vi "Tmp_M submodule.vi"(9 "timeout ms":i32=1000) -> (0 "Error Out":errorcluster, 3 "Temperatures":T2[](array[typedef]) {"Time stamp" format="%<%H:%M:%S%2u\n%Y/%m/%d>T"})   [LabVIEW 2021, in "Temperature monitor.lvlib"]
doc: "Magnet module controls: power supply unit (PSU/SMS) and temperature monitor (TM/LSC218).\nPSU controls mainly: switch heater and ramping of current which runs throught coil.\nTM controls temperature of switch, coil and cryostat.\nMessage for magnet is a cluster that contains: {(enum) Command , (variant) Data}\nFor simplifieing of documentation, the Command is noted as a name of instruction, and Data is represented by a requered datatype (mostly cluster) name.\nCommands:\nInitialize(Magnet Config Constants) - Sugesstion: Load configuration constants from configuration file.\nSet field (Set field{B, R, cr}) - B-field[T], R-ramp[A/s], cr - custom ramp[bool].\nSwitch mode(mode) - to persistant, or to ramping.\nBlackout() - undone functionality of emergency deenergizing.\nUpdate() - Important! This triggers update of data from instruments. Shoud occure in regular intervals as priority message.\nResponses:\nMagnet initialized ();\nTM revision(temperature monitor revision);\nMagnet init error(error);\nSetting field(Set Field{B, R, cr});\nWarning(string);\nSwitching to(mode);\nUpdate error(error);\nTM update(TM sensors);\nPSU update(PSU data);\nMagnet status();"
uses:
  submodules/Temperature monitor/Temperature monitor.lvlib
  ctl/Cryostat temperature sensors.ctl
  Magnet module.lvlib
  Messenger service/Data types/Module name.ctl
  Messenger service/MessengerLib.lvlib
  ctl/TM states.ctl
  <userlib>/Queued messenger lib/Queued messenger.lvlib
  <userlib>/Queued messenger lib/TypeDefs/Mailbox ref.ctl
  submodules/Temperature monitor/Typedefs/TM_status.ctl
  <vilib>/WebDAVClient/NI_WebDAV.lvlib
panel:
  in  "Instr VISA ref":refnum<visa-resource-name>
  in  "This mailbox":T1
  in  "Supra mailbox":T1
  out "Connected":bool
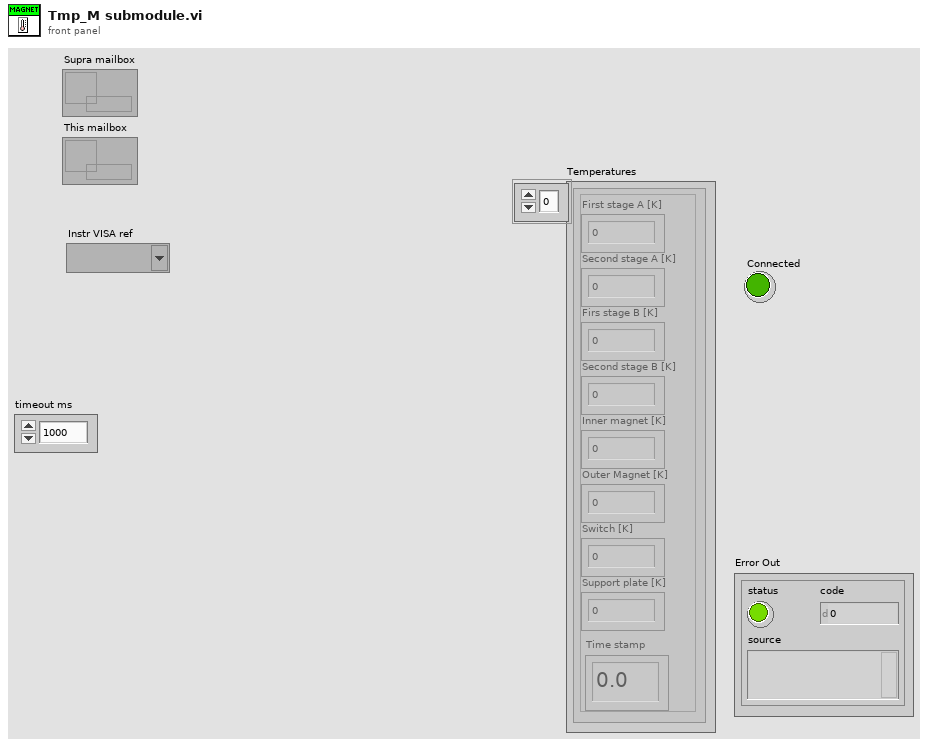
[diagram p1: front panel]
types:
  T1 = typedef "Queued messenger.lvlib/Mailbox ref.ctl" = refnum<queue>
  T2 = typedef "Magnet module.lvlib/Cryostat temperature sensors.ctl" = cluster{"First stage A [K]":dbl, "Second stage A [K]":dbl, "Firs stage B [K]":dbl, "Second stage B [K]":dbl, "Inner magnet [K]":dbl, "Outer Magnet [K]":dbl, "Switch [K]":dbl, "Support plate [K]":dbl, "Time stamp":dbl}
  T3 = typedef "TM_status.ctl" = cluster{"Supramodule":T1, "This module":T1, "Standalone?":bool, "Stopped?":bool, "Instr VISA ref":refnum<visa-resource-name>, "Connected?":bool}
  T4 = typedef "TM states.ctl" = enum16{"Initialize", "Wait for event", "Check message", "End"}
  T5 = typedef "MessengerLib.lvlib/Module name.ctl" = enum16{"Emty", "Magnet", "VTI", "Excitation", "Servo", "Acquisition", "Rotator", "Digitizer", "SMU2450", "Carousel", "Multimeter", "Tmp monitor", "Power monitor"}
  T6 = enum32{"Bad", "Idle", "Run top level", "Running"}
  T7 = typedef "Temperature monitor.lvlib/Tmp_M commands.ctl" = enum16{"Ignore", "Connect", "Set timeout", "Update", "Disconnect"}
  T8 = typedef "MessengerLib.lvlib/Mailbox address.ctl" = refnum<queue>
  T9 = typedef "Temperature monitor.lvlib/TM Revision.ctl" = cluster{"Instr Serial Number":string, "Instr Driver Revision":string, "Instr Firmware Revision":string, "Instr Model Number":string}
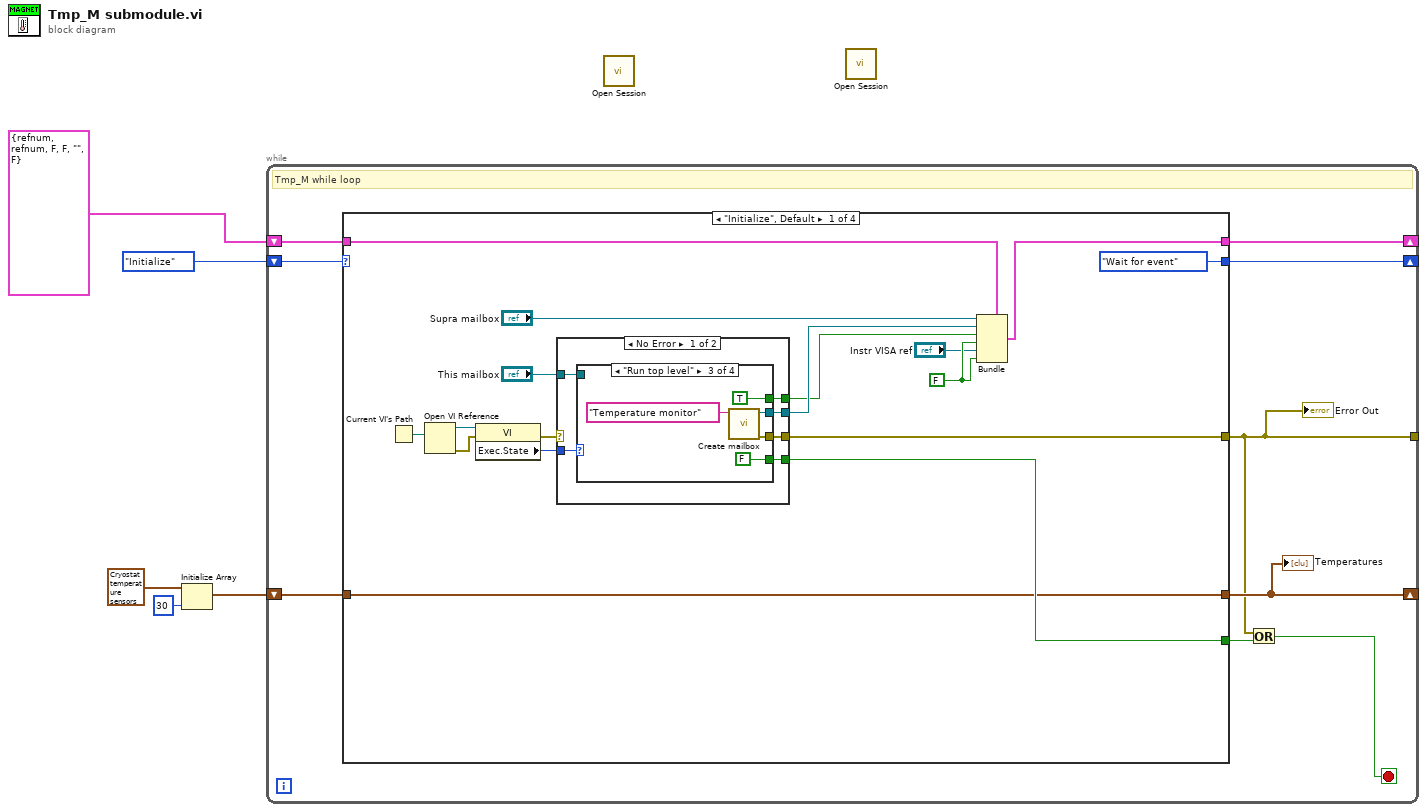
[diagram p0: block diagram]
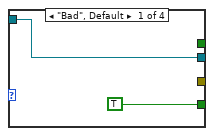
[diagram p2: hidden frame]
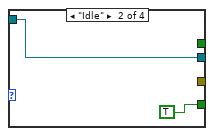
[diagram p3: hidden frame]
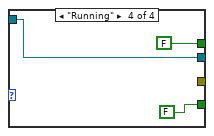
[diagram p4: hidden frame]
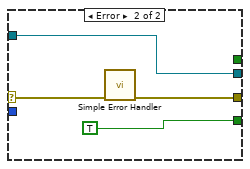
[diagram p5: hidden frame]
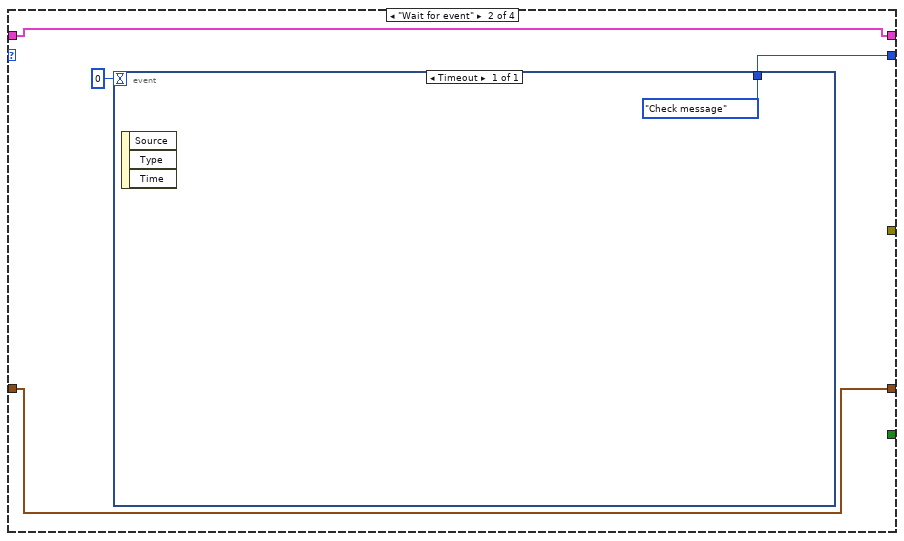
[diagram p6: hidden frame]
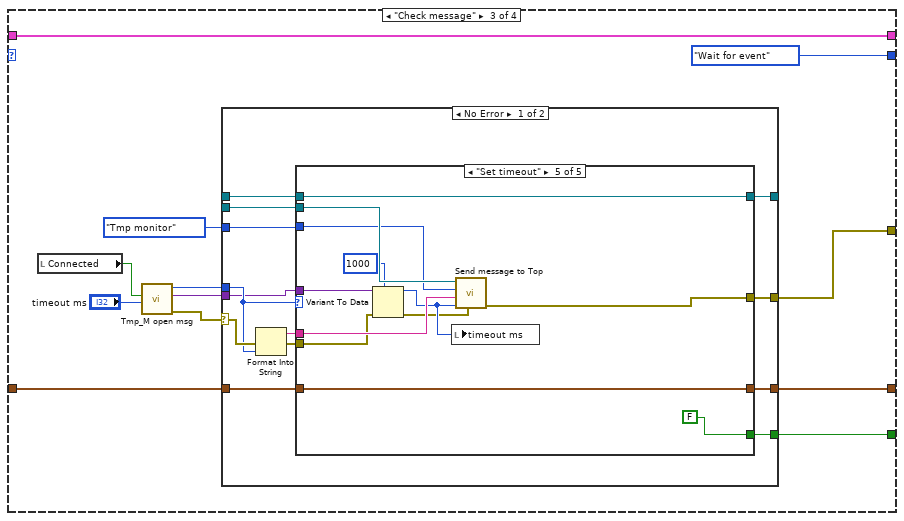
[diagram p7: hidden frame]
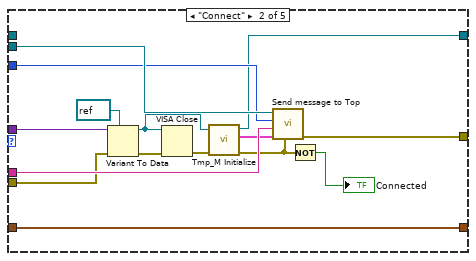
[diagram p9: hidden frame]
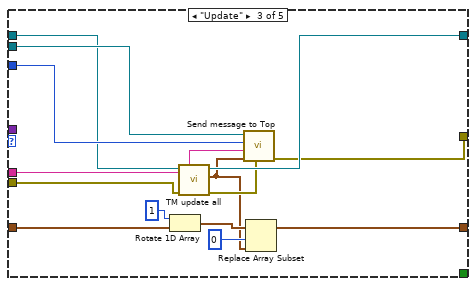
[diagram p10: hidden frame]
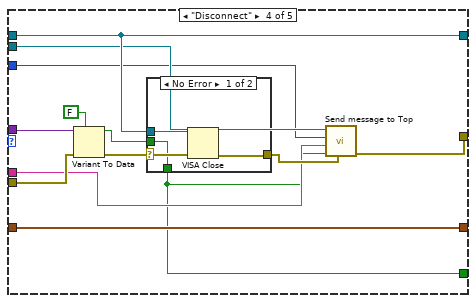
[diagram p11: hidden frame]
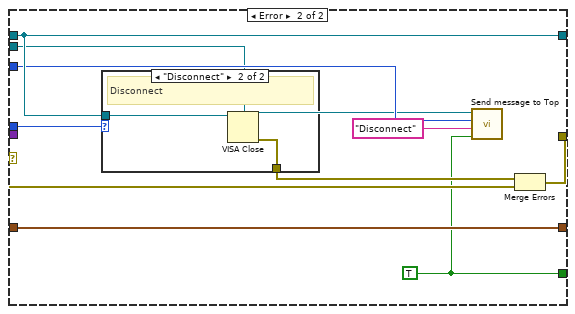
[diagram p13: hidden frame]
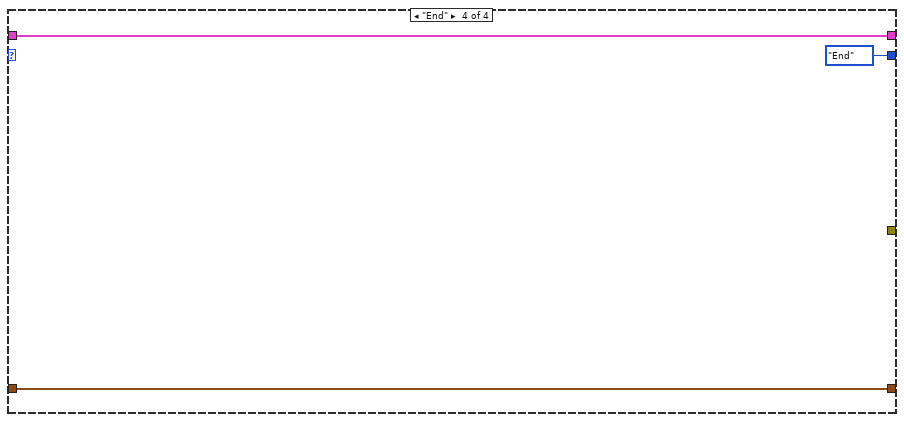
[diagram p15: hidden frame]
diagram:
  n1 = Initialize Array(T2 {"First stage A [K]"=0.0, "Second stage A [K]"=0.0, "Firs stage B [K]"=0.0, "Second stage B [K]"=0.0, "Inner magnet [K]"=0.0, "Outer Magnet [K]"=0.0, "Switch [K]"=0.0, "Support plate [K]"=0.0, "Time stamp"=0.0} ("LSC218 sensors"), 30 ("dimension size")) -> (w5:T2[])
  n2 = while {
    shift-right: [w13] -> _
    shift-left: w5 -> [w14]
    tunnel: [w7] -> _
    shift-right: [w10] -> _
    shift-left: TM_states."Initialize" -> [w11]
    shift-right: [w6] -> _
    shift-left: T3 {"Supramodule"=refnum, "This module"=refnum, "Standalone?"=FALSE, "Stopped?"=FALSE, "Instr VISA ref"="", "Connected?"=FALSE} ("Temperature monitor status") -> [w9]
    stop <- w8 stop-if-true
    # "Tmp_M while loop"
    n3 = case shown="\"Initialize\", Default" w11 {
      tunnel: w14 -> [w17 w54 w73 w162]
      tunnel: [w17 w54 w72 w162] -> w13
      tunnel: [w25 _ w65 _] -> w12
      tunnel: [w23 _ w61 _] -> w7
      tunnel: [TM_states."Wait for event" w57 TM_states."Wait for event" TM_states."End"] -> w10
      tunnel: w9 -> [w24 w55 w59 w163]
      tunnel: [w18 w55 w59 w163] -> w6
      frame "Initialize", Default {
        w20 = FALSE ("Connected?")
        n4 = Current VI's Path() -> (path=w29:path)
        n5 = Open VI Reference(vi path=w29) -> (vi reference=w30:refnum<vi>, error out=w28:errorcluster)  [unwired: 5 in]
        n6 = property class="VI"(reference=w30, error in=w28) -> (error out=w26:errorcluster, "Exec.State"=w27:T6)  [unwired: 1 out]
        n7 = case shown="No Error" w26 {
          selector: w26 -> [_ w52]
          tunnel: w27 -> [w37 _]
          tunnel: [w36 TRUE] -> w25
          tunnel: [w35 w51] -> w22
          tunnel: "This mailbox" -> [w34 w51]
          tunnel: [w33 _] -> w21
          tunnel: [w32 w50] -> w23
          frame No Error {
            n8 = case shown="\"Run top level\"" w37 {
              tunnel: [TRUE TRUE FALSE FALSE] -> w36
              tunnel: [w38 w40 w44 w48] -> w35
              tunnel: w34 -> [w38 w40 _ w48]
              tunnel: [_ _ TRUE FALSE] -> w33
              tunnel: [_ _ w42 _] -> w32
              frame "Bad", Default {
              }
              frame "Idle" {
              }
              frame "Run top level" {
                n9 = call <userlib>:"Create mailbox.vi"("name (unnamed)"="Temperature monitor") -> ("error out"=w42:errorcluster, "Mailbox ref"=w44:T1)  [unwired: 4 in, 1 out]
              }
              frame "Running" {
              }
            }
          }
          frame Error {
            n10 = call <vilib>:"Simple Error Handler.vi"("error in (no error)"=w52) -> ("error out"=w50:errorcluster)  [unwired: 4 in, 4 out]
          }
        }
        n11 = Bundle(cluster=w24, "Supramodule"="Supra mailbox", "This module"=w22, "Standalone?"=w21, "Stopped?"=w20, "Instr VISA ref"="Instr VISA ref", "Connected?"=w20) -> (w18:T3)
      }
      frame "Wait for event" {
        n12 = event shown="[0] Timeout" {
          selector: _ -> [_]
          dyn-events: _ -> [_]
          timeout: 0 -> [_]
          tunnel: [TM_states."Check message"] -> w57
          event Timeout {
            n13 = event-data() -> ()  [unwired: 1 in, 3 out]
          }
        }
      }
      frame "Check message" {
        n14 = local read "Connected"() -> (w62:bool)
        n15 = call "Tmp_M open msg.vi"("timeout ms (1000)"="timeout ms", "Connected"=w62) -> ("error out"=w67:errorcluster, "Data"=w66:variant, "Command"=w68:T7, "Queue in"=w69:T8)  [unwired: 4 in, 2 out]
        n16 = case shown="No Error" w67 {
          selector: w67 -> [w80 w154]
          tunnel: [w87 w152] -> w74
          tunnel: w68 -> [w79 w158]
          tunnel: w73 -> [w86 w159]
          tunnel: [w85 w159] -> w72
          tunnel: [w76 w150] -> w65
          tunnel: [w83 w157] -> w71
          tunnel: [w82 w157] -> w70
          tunnel: w66 -> [w78 _]
          tunnel: [w77 w156] -> w61
          tunnel: Module_name."Tmp monitor" ("Module") -> [w75 w153]
          frame No Error {
            n17 = Format Into String(error in=w80, w79) -> (resulting string=w84:string, error out=w81:errorcluster)  [unwired: 2 in]
            n18 = case shown="\"Set timeout\"" w79 {
              tunnel: w87 -> [_ w105 w115 w124 w148]
              tunnel: w86 -> [w90 w104 w119 w132 w149]
              tunnel: [w90 w104 w118 w132 w149] -> w85
              tunnel: w75 -> [_ w101 w116 w123 w145]
              tunnel: w84 -> [_ w102 w117 w122 w146]
              tunnel: [_ _ _ w120 FALSE] -> w76
              tunnel: [w89 w98 w113 w131 w144] -> w83
              tunnel: w82 -> [w89 _ w114 w131 w144]
              tunnel: w81 -> [w88 w94 w106 w128 w141]
              tunnel: w78 -> [_ w93 _ w129 w142]
              tunnel: [w88 w92 w112 w125 w138] -> w77
              frame "Ignore", Default {
              }
              frame "Connect" {
                n19 = Variant To Data(error in=w94, type=refnum<visa-resource-name> refnum ("LSC218"), Variant=w93) -> (data=w97:refnum<visa-resource-name>, error out=w103:errorcluster)
                n20 = VISA Close(VISA resource name=w97, error in (no error)=w103) -> (error out=w100:errorcluster)
                n21 = call "Tmp_M Initialize.vi"("error in (no error)"=w100, "VISA Refnum in"=w97) -> ("error out"=w95:errorcluster, "TM Revision"=w99:T9, "VISA Refnum out"=w98:refnum<visa-resource-name>)  [unwired: 7 in]
                n22 = call "Send message to Top.vi"("Error in (no error)"=w95, "Data"=w99, "Response"=w102, "Module"=w101, "Mailbox address in"=w105) -> ("Error out"=w92:errorcluster)  [unwired: 5 in, 1 out]
                n23 = Not(x=w95) -> (.not. x?=→"Connected":bool)
              }
              frame "Update" {
                n24 = Rotate 1D Array(1:w119, 2:1 ("n")) -> (0:w110:T2[])
                n25 = call "TM update all.vi"("error in (no error)"=w106, "VISA Refnum in"=w114) -> ("error out"=w108:errorcluster, "LSC218 sensors"=w107:T2, "VISA Refnum out"=w113:refnum<visa-resource-name>)  [unwired: 7 in]
                n26 = call "Send message to Top.vi"("Error in (no error)"=w108, "Data"=w107, "Response"=w117, "Module"=w116, "Mailbox address in"=w115) -> ("Error out"=w112:errorcluster)  [unwired: 5 in, 1 out]
                n27 = Replace Array Subset(array=w110, new element=w107, index=0) -> (w118:T2[])
              }
              frame "Disconnect" {
                n28 = Variant To Data(error in=w128, type=FALSE, Variant=w129) -> (data=w121:bool, error out=w127:errorcluster)
                n29 = case shown="No Error" w127 {
                  selector: w127 -> [w135 w137]
                  tunnel: w131 -> [w136 _]
                  tunnel: [w134 w137] -> w126
                  tunnel: w121 -> [w133 _]
                  tunnel: [w133 _] -> w120
                  frame No Error {
                    n30 = VISA Close(VISA resource name=w136, error in (no error)=w135) -> (error out=w134:errorcluster)
                  }
                  frame Error {
                  }
                }
                n31 = call "Send message to Top.vi"("Error in (no error)"=w126, "Data"=w120, "Response"=w122, "Module"=w123, "Mailbox address in"=w124) -> ("Error out"=w125:errorcluster)  [unwired: 5 in, 1 out]
              }
              frame "Set timeout" {
                n32 = Variant To Data(error in=w141, type=1000 ("timeout ms"), Variant=w142) -> (data=w140:i32, error out=w139:errorcluster)
                n33 = local write "timeout ms"(w140) -> ()
                n34 = call "Send message to Top.vi"("Error in (no error)"=w139, "Data"=w140, "Response"=w146, "Module"=w145, "Mailbox address in"=w148) -> ("Error out"=w138:errorcluster)  [unwired: 5 in, 1 out]
              }
            }
          }
          frame Error {
            w150 = TRUE
            n35 = case shown="\"Disconnect\"" w158 {
              tunnel: w157 -> [_ w161]
              tunnel: [_ w160] -> w155
              frame "Ignore", Default {
                # "Nohing"
              }
              frame "Disconnect" {
                # "Disconnect"
                n36 = VISA Close(VISA resource name=w161) -> (error out=w160:errorcluster)  [unwired: 1 in]
              }
            }
            n37 = call "Send message to Top.vi"("Data"=w150, "Response"="Disconnect", "Module"=w153, "Mailbox address in"=w152) -> ()  [unwired: 6 in, 2 out]
            n38 = Merge Errors(w155, w154) -> (w156:errorcluster)
          }
        }
      }
      frame "End" {
      }
    }
    "Temperatures" <- w13
    "Error Out" <- w7
    n39 = Or(x=w7, y=w12) -> (x .or. y?=w8:bool)
  }
  n40 = call <vilib>:"Open Session.vi"() -> ()  [unwired: 14 in, 2 out]
  n41 = call <vilib>:"Open Session.vi"() -> ()  [unwired: 14 in, 2 out]
